vi "Linhas XY-trigger.vi"() -> ()   [LabVIEW 2016]
doc: "André Romero - 2023\nandretec@ifsc.usp.br\nIFSC - USP"
panel:
  in  "stop":bool
  out "Progress":i32=56
  out "Stop":bool
  in  "Acc":dbl=0.45
  in  "Velocity":sgl=0.45
  out "Motor M1":bool=TRUE
  out "Motor M2":bool=TRUE
  in  "Swap motor":bool
  in  "d (um)":dbl=1.0
  in  "L (um)":dbl=500.0
  in  "N Lines":i32=100
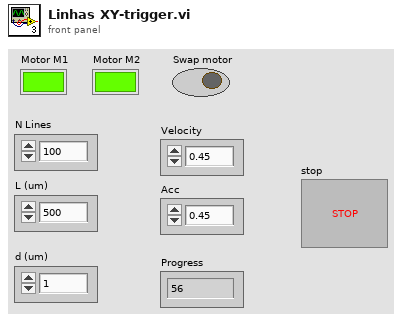
[diagram p1: front panel]
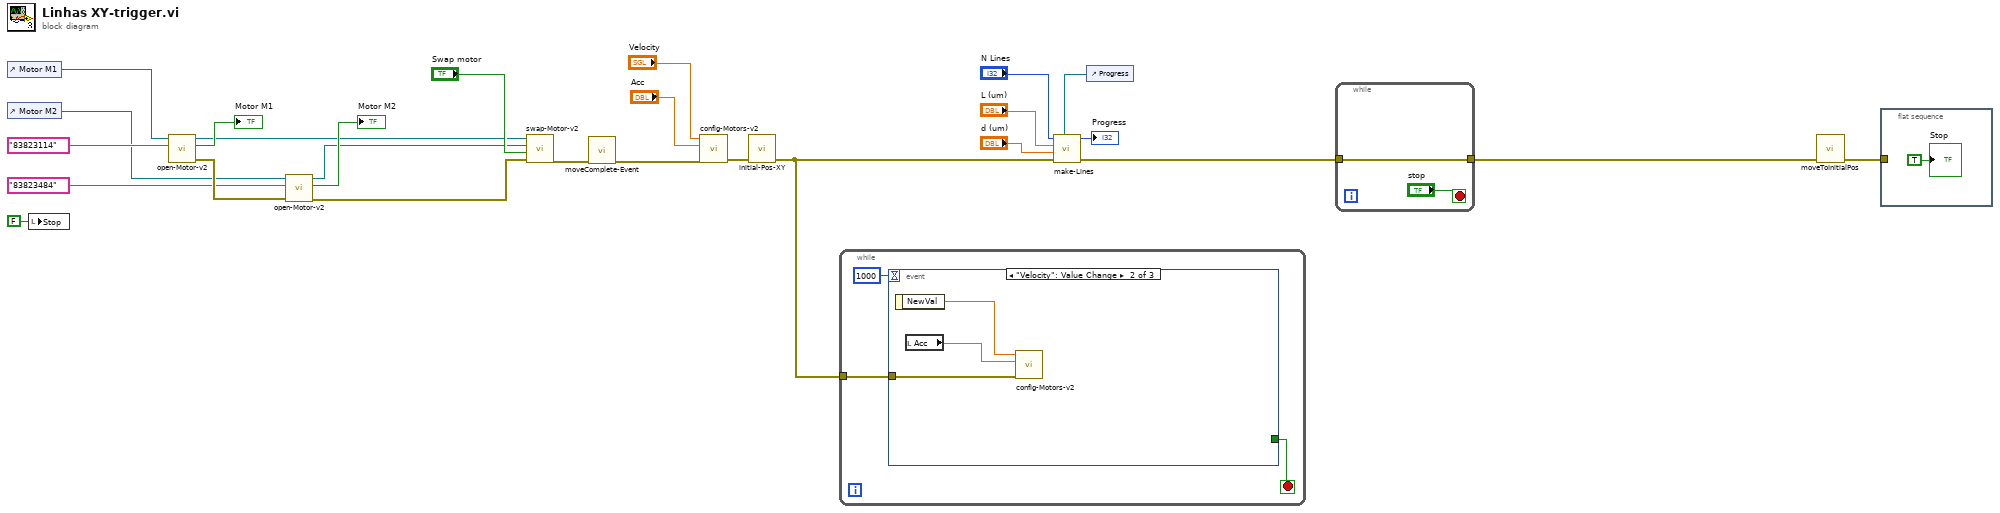
[diagram p0: block diagram]
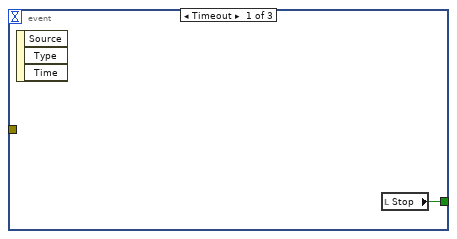
[diagram p2: hidden frame]
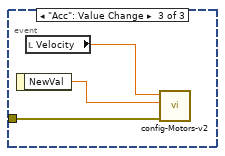
[diagram p3: hidden frame]
diagram:
  n1 = control-ref of="Motor M1"() -> (w20:refnum<vi>)
  n2 = control-ref of="Motor M2"() -> (w19:refnum<vi>)
  n3 = local write "Stop"(FALSE ("Stop")) -> ()
  n4 = call "open-Motor-v2.vi"("S/N Motor"="83823114", "ref Boolean in"=w20) -> ("Error Out"=w26:errorcluster, "Motor Status"=→"Motor M1":bool, "Refnum out"=w2:refnum<k7>)  [unwired: 7 in]
  n5 = call "open-Motor-v2.vi"("Error In"=w26, "S/N Motor"="83823484", "ref Boolean in"=w19) -> ("Error Out"=w18:errorcluster, "Motor Status"=→"Motor M2":bool, "Refnum out"=w1:refnum<k7>)  [unwired: 6 in]
  n6 = call "swap-Motor-v2.vi"("error in (no error)"=w18, "Swap motor"="Swap motor", "Refnum in M2"=w1, "Refnum in M1"=w2) -> ("error out"=w15:errorcluster)  [unwired: 7 in]
  n7 = call "moveComplete-Event.vi"("Error In"=w15) -> ("Error Out"=w14:errorcluster)  [unwired: 10 in]
  n8 = call "config-Motors-v2.vi"("error in"=w14, "Acc"="Acc", "Velocity"="Velocity") -> ("error out"=w9:errorcluster)  [unwired: 8 in]
  n9 = call "initial-Pos-XY.vi"("error in (no error)"=w9) -> ("error out"=w8:errorcluster)  [unwired: 10 in]
  n10 = while {
    tunnel: w8 -> [w27]
    stop <- w28 stop-if-true
    n11 = event shown="[1] \"Velocity\": Value Change" {
      selector: _ -> [_ _ _]
      dyn-events: _ -> [_ _ _]
      timeout: 1000 -> [_ _ _]
      tunnel: [w30 _ _] -> w28
      tunnel: w27 -> [_ w33 w36]
      event Timeout {
        n12 = event-data() -> ()  [unwired: 1 in, 3 out]
        n13 = local read "Stop"() -> (w30:bool)
      }
      event "Velocity": Value Change {
        n14 = event-data() -> ("NewVal"=w32:sgl)  [unwired: 1 in]
        n15 = local read "Acc"() -> (w31:dbl)
        n16 = call "config-Motors-v2.vi"("error in"=w33, "Acc"=w31, "Velocity"=w32) -> ()  [unwired: 8 in, 1 out]
      }
      event "Acc": Value Change {
        n17 = event-data() -> ("NewVal"=w34:dbl)  [unwired: 1 in]
        n18 = local read "Velocity"() -> (w35:sgl)
        n19 = call "config-Motors-v2.vi"("error in"=w36, "Acc"=w34, "Velocity"=w35) -> ()  [unwired: 8 in, 1 out]
      }
    }
  }
  n20 = control-ref of="Progress"() -> (w3:refnum<vi>)
  n21 = call "make-Lines.vi"("Progress"=w3, "error in"=w8, "d (um)"="d (um)", "L (um)"="L (um)", "N Lines"="N Lines") -> ("error out"=w7:errorcluster, "Progress"=→"Progress":i32)  [unwired: 5 in]
  n22 = while {
    tunnel: w7 -> [w37]
    tunnel: [w37] -> w6
    stop <- "stop" stop-if-true
  }
  n23 = call "moveToInitialPos.vi"("error in (no error)"=w6) -> ("error out"=w5:errorcluster)  [unwired: 10 in]
  n24 = flat-sequence {
    tunnel: w5 -> [_]
    frame #0 {
      "Stop" <- TRUE ("Stop")
    }
  }
